vi "update_vfile.vi"(8 "error in":errorcluster, 10 "Vfile (V)":variant, 11 "Channel":T1={" Card.Channel"=1.12, "Crate"=0} {"Card.Channel" format="%.2f"}) -> (0 "error out":errorcluster)   [LabVIEW 2018]
uses:
  channel_cluster.ctl
  channel.ctl
  CAEN globals.vi
panel:
  out "Updated Channel Array Val":T2[](array[typedef]) {"Vfile (V)" format="%.1f V"; "Vswmax (V)" format="%#_g V"; "Iset (A)" format="%.2pA"; "Imon (A)" format="%.2pA"; "Vset (V)" format="%#_g V"; "Vmon (V)" format="%.1f V"}
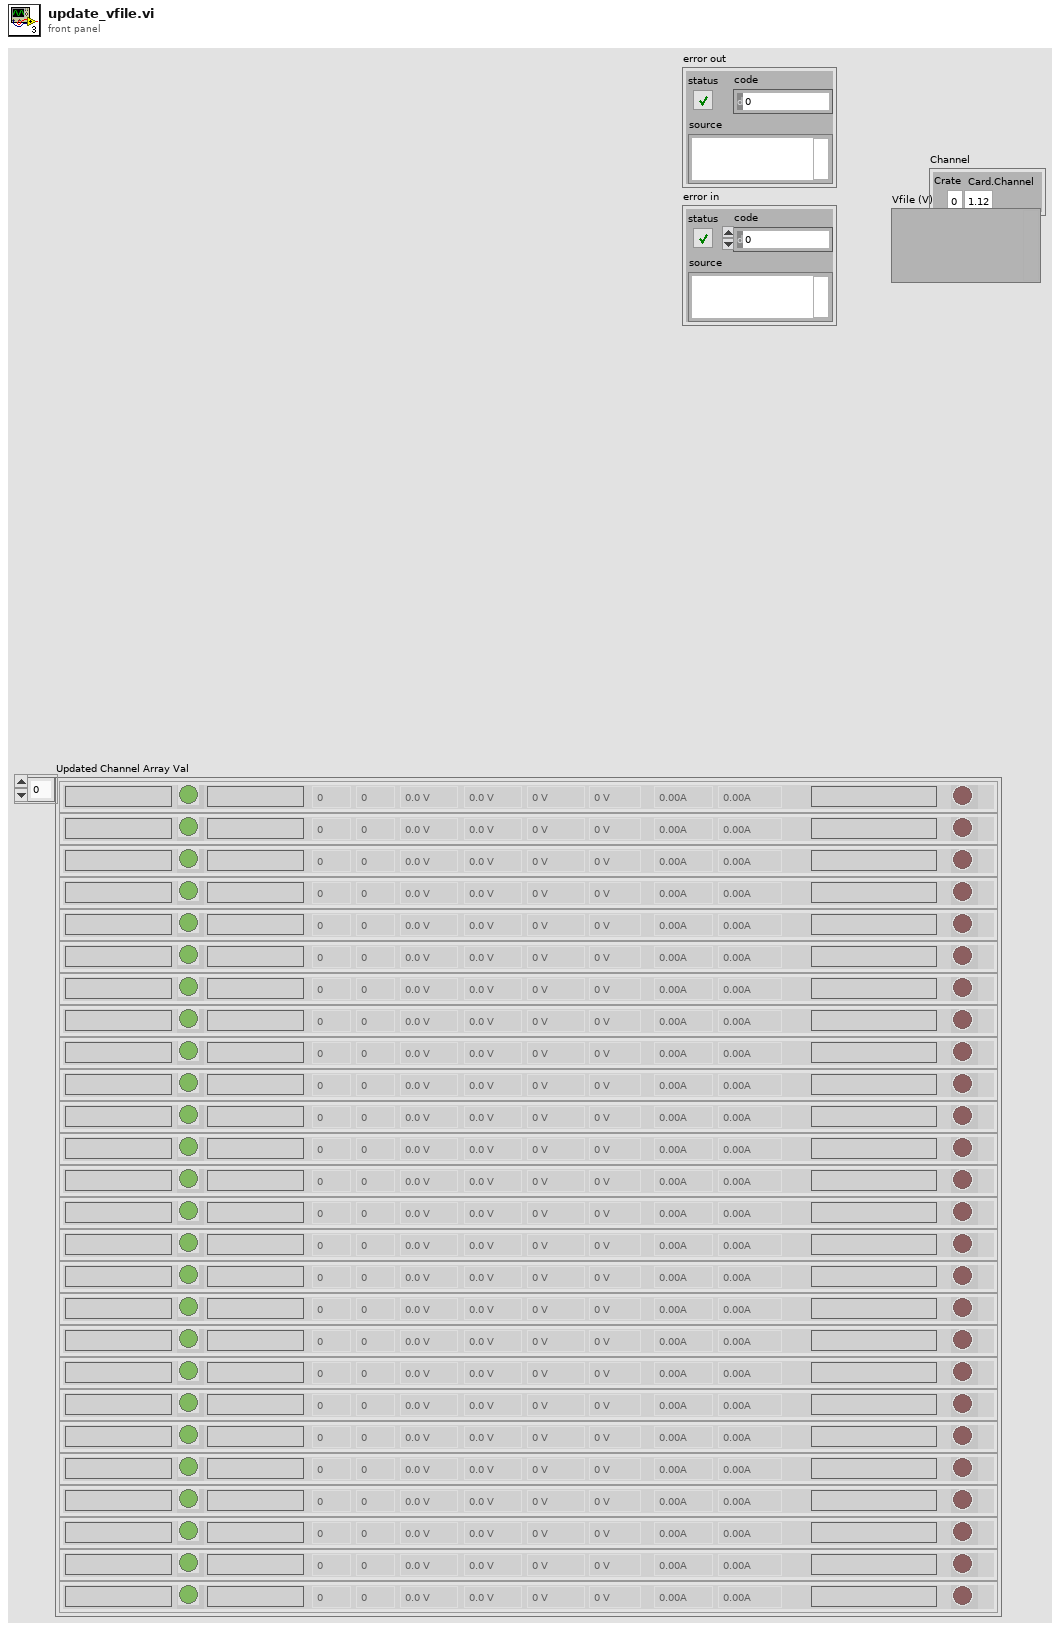
[diagram p1: front panel]
types:
  T1 = typedef "channel.ctl" = cluster{" Card.Channel":dbl, "Crate":i32}
  T2 = typedef "channel_cluster.ctl" = cluster{"Channel Name":string, "Crate":i32, "Card Type":string, "Card":i32, "Channel":i32, "Status Icon":picture, "Vmon (V)":dbl, "Vset (V)":dbl, "Imon (A)":dbl, "Iset (A)":dbl, "Timestamp":string, "ON/OFF":bool, "Status":string, "Vswmax (V)":dbl, "Flag":bool, "Vfile (V)":dbl, "Error Logged":bool[], "enable_file":bool}
  T3 = cluster{"Group Name":string, "Channels in Group":T1[]}[]
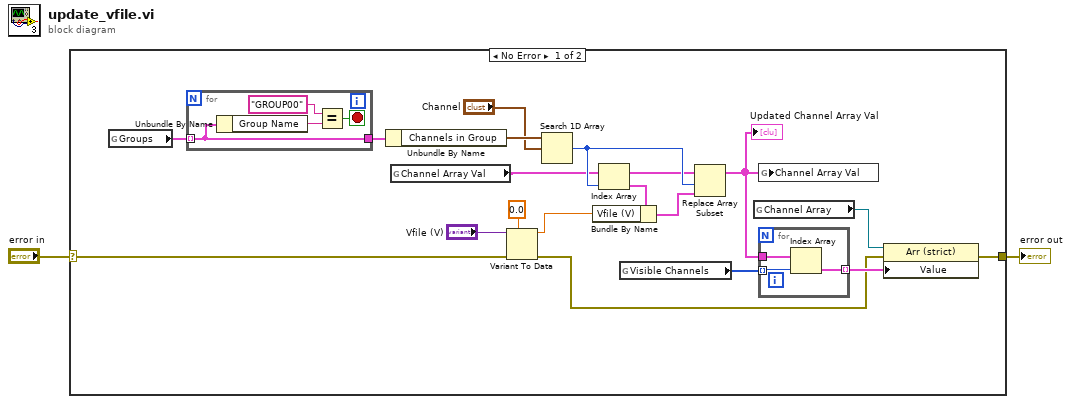
[diagram p0: block diagram]
diagram:
  n1 = case shown="No Error" "error in" {
    selector: "error in" -> [w4 w28]
    tunnel: [w8 w28] -> w2
    frame No Error {
      n2 = global read "CAEN globals.vi" "Groups"() -> (w17:T3)
      n3 = for {
        tunnel: w17 -> [w25] mode=indexing
        tunnel: [w25] -> w18
        stop <- w24 stop-if-true
        n4 = Unbundle By Name(w25) -> ("Group Name"=w27:string)
        n5 = Equal?(x="GROUP00" ("Group Name"), y=w27) -> (x = y?=w24:bool)
      }
      n6 = Unbundle By Name(w18) -> ("Channels in Group"=w16:T1[])
      n7 = global read "CAEN globals.vi" "Channel Array Val"() -> (w15:T2[])
      n8 = Variant To Data(error in=w4, type=0.0 ("Vfile (V)"), Variant="Vfile (V)") -> (data=w6:dbl, error out=w5:errorcluster)
      n9 = Search 1D Array(1D array=w16, element="Channel") -> (index of element=w20:i32)  [unwired: 1 in]
      n10 = Index Array(array=w15, index=w20) -> (element=w10:T2)
      n11 = Bundle By Name(cluster=w10, "Vfile (V)"=w6) -> (w19:T2)
      n12 = global read "CAEN globals.vi" "Visible Channels"() -> (w14:i32[])
      n13 = Replace Array Subset(array=w15, new element=w19, index=w20) -> (w11:T2[])
      "Updated Channel Array Val" <- w11
      n14 = global read "CAEN globals.vi" "Channel Array"() -> (w13:refnum<vi>)
      n15 = global write "CAEN globals.vi" "Channel Array Val"(w11) -> ()
      n16 = for {
        tunnel: w14 -> [w22] mode=indexing
        tunnel: w11 -> [w23]
        tunnel: [w21] -> w12 mode=indexing
        n17 = Index Array(array=w23, index=w22) -> (element=w21:T2)
      }
      n18 = property class="Arr (strict)"(reference=w13, error in=w5, "Value"=w12) -> (error out=w8:errorcluster)  [unwired: 1 out]
    }
    frame Error {
    }
  }
  "error out" <- w2
